vi "Shutdown Frame Grabber.vi"(8 "error in (no error)":errorcluster, 10 "Frame grabber connected?":bool, 11 "Frame Grabber Data in":T1={"Camera Session"="", "Frame"=refnum, "AVI Refnum"=refnum, "Codecs"=[], "Frame number"=0, "Tracking File Refnum"=refnum, "Tick Count"=0, "Probe Object"=refnum, "Playback Probe Data"=[], "Rigid Body"={"Position"={"x (mm)"=0.0, "y (mm)"=0.0, "z (mm)"=0.0}, "Orientation"={"Pitch (rad)"=0.0, "Yaw (rad)"=0.0, "Roll (rad)"=0.0}, "Quaternion"={"qx"=0.0, "qy"=0.0, "qz"=0.0, "qw"=0.0}, "Tracked?"=FALSE}, "Total no frames playback"=0, "Video FPS"=0.0, "Camera connected?"=FALSE, "Scene"=refnum, "Cropped Frame"=refnum, "Tracker FPS"=0.0, "Crop ROI"=[], "Presentation Values"=[], "Elapsed time (ms)"=0, "Camera frames playback"=0, "Refnums"={"Live Refnum"=refnum, "Record Refnum"=refnum, "Recording Settings Refnum"=refnum, "Playback Refnum"=refnum, "Frame Slider Refnum"=refnum, "Pause Refnum"=refnum, "Home Refnum"=refnum, "Crop Refnum"=refnum, "Clear Crop Refnum"=refnum, "stop refnum"=refnum, "Playback Rate Refnum"=refnum, "Operator Settings Refnums"=refnum, "Presentation Refnum"=refnum, "Gestation Refnum"=refnum, "Connection Settings Refnum"=refnum, "Crop Time Frame Slider Refnum"=refnum, "Cancel Save Refnum"=refnum, "Reverse Playback Refnum"=refnum}, "Dimensions"={"Probe Dimensions"={"Probe Width"=0.0, "Probe Depth"=1.0, "Probe Height"=0.0}, "Room Dimensions"={"Room Width"=0.0, "Room Depth"=0.0, "Room Height"=0.0}}, "Playback Data As Strings"=[], "Cropped Tracking File Refnum"=refnum, "Cropped AVI Refnum"=refnum, "Header"=[], "Total euclidian distance"=0.0}) -> (0 "error out":errorcluster, 2 "Disconnect":bool, 3 "Frame Grabber Data out":T1={"Camera Session"="", "Frame"=refnum, "AVI Refnum"=refnum, "Codecs"=[], "Frame number"=0, "Tracking File Refnum"=refnum, "Tick Count"=0, "Probe Object"=refnum, "Playback Probe Data"=[], "Rigid Body"={"Position"={"x (mm)"=0.0, "y (mm)"=0.0, "z (mm)"=0.0}, "Orientation"={"Pitch (rad)"=0.0, "Yaw (rad)"=0.0, "Roll (rad)"=0.0}, "Quaternion"={"qx"=0.0, "qy"=0.0, "qz"=0.0, "qw"=0.0}, "Tracked?"=FALSE}, "Total no frames playback"=0, "Video FPS"=0.0, "Camera connected?"=FALSE, "Scene"=refnum, "Cropped Frame"=refnum, "Tracker FPS"=0.0, "Crop ROI"=[], "Presentation Values"=[], "Elapsed time (ms)"=0, "Camera frames playback"=0, "Refnums"={"Live Refnum"=refnum, "Record Refnum"=refnum, "Recording Settings Refnum"=refnum, "Playback Refnum"=refnum, "Frame Slider Refnum"=refnum, "Pause Refnum"=refnum, "Home Refnum"=refnum, "Crop Refnum"=refnum, "Clear Crop Refnum"=refnum, "stop refnum"=refnum, "Playback Rate Refnum"=refnum, "Operator Settings Refnums"=refnum, "Presentation Refnum"=refnum, "Gestation Refnum"=refnum, "Connection Settings Refnum"=refnum, "Crop Time Frame Slider Refnum"=refnum, "Cancel Save Refnum"=refnum, "Reverse Playback Refnum"=refnum}, "Dimensions"={"Probe Dimensions"={"Probe Width"=0.0, "Probe Depth"=1.0, "Probe Height"=0.0}, "Room Dimensions"={"Room Width"=0.0, "Room Depth"=0.0, "Room Height"=0.0}}, "Playback Data As Strings"=[], "Cropped Tracking File Refnum"=refnum, "Cropped AVI Refnum"=refnum, "Header"=[], "Total euclidian distance"=0.0})   [LabVIEW 2017]
uses:
  Controls/Frame Grabber Data.ctl
  <vilib>/userdefined/High Color/IMAQdx.ctl
  <vilib>/vision/Image Controls.llb/IMAQ Image.ctl
  <vilib>/vision/Avi.llb/IMAQ AVI2 Refnum.ctl
  Controls/Rigid Body Info.ctl
  Controls/Position.ctl
  Controls/Orientation.ctl
  Controls/Refnums.ctl
  Controls/Recording Settings.ctl
  Controls/Operator Settings.ctl
  Controls/Operator.ctl
  Controls/Dimensions.ctl
  Controls/Room Dimensions.ctl
  <vilib>/vision/driver/NI_Vision_Acquisition_Software.lvlib
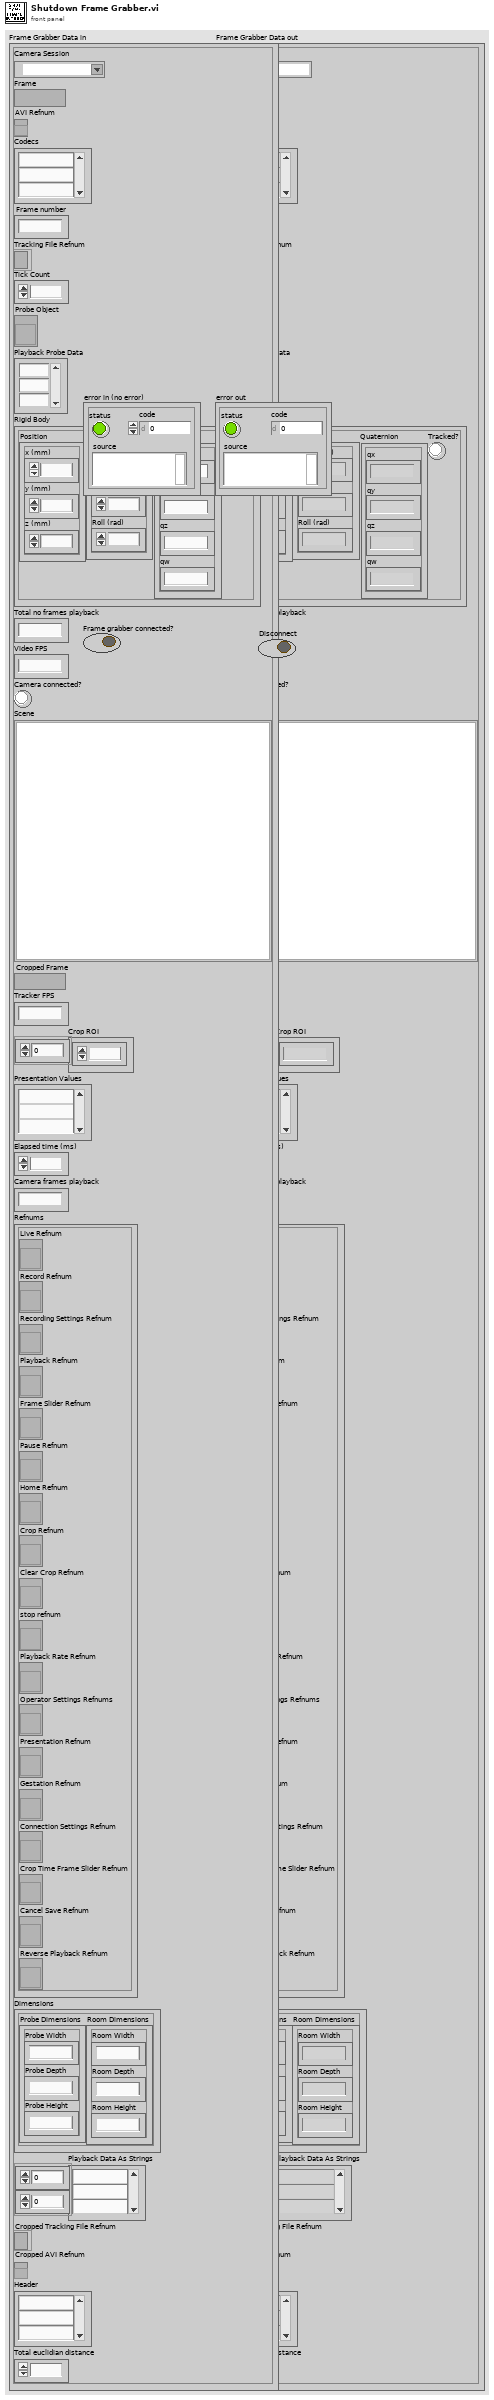
[diagram p1: front panel]
types:
  T1 = typedef "Frame Grabber Data.ctl" = cluster{"Camera Session":T2, "Frame":T3, "AVI Refnum":T4, "Codecs":string[], "Frame number":u32, "Tracking File Refnum":refnum<file>, "Tick Count":u32, "Probe Object":refnum<vi>, "Playback Probe Data":dbl[][], "Rigid Body":T5, "Total no frames playback":i32, "Video FPS":dbl, "Camera connected?":bool, "Scene":refnum<vi>, "Cropped Frame":T3, "Tracker FPS":dbl, "Crop ROI":i32[], "Presentation Values":string[], "Elapsed time (ms)":u32, "Camera frames playback":u32, "Refnums":T8, "Dimensions":T9, "Playback Data As Strings":string[][], "Cropped Tracking File Refnum":refnum<file>, "Cropped AVI Refnum":T4, "Header":string[], "Total euclidian distance":dbl}
  T2 = typedef "IMAQdx.ctl" = refnum<k21>
  T3 = typedef "IMAQ Image.ctl" = refnum<image>
  T4 = typedef "IMAQ AVI2 Refnum.ctl" = refnum<k20>
  T5 = typedef "Rigid Body Info.ctl" = cluster{"Position":T6, "Orientation":T7, "Quaternion":cluster{"qx":sgl, "qy":sgl, "qz":sgl, "qw":sgl}, "Tracked?":bool}
  T6 = typedef "Position.ctl" = cluster{"x (mm)":sgl, "y (mm)":sgl, "z (mm)":sgl}
  T7 = typedef "Orientation.ctl" = cluster{"Pitch (rad)":sgl, "Yaw (rad)":sgl, "Roll (rad)":sgl}
  T8 = typedef "Refnums.ctl" = cluster{"Live Refnum":refnum<vi>, "Record Refnum":refnum<vi>, "Recording Settings Refnum":refnum<vi>, "Playback Refnum":refnum<vi>, "Frame Slider Refnum":refnum<vi>, "Pause Refnum":refnum<vi>, "Home Refnum":refnum<vi>, "Crop Refnum":refnum<vi>, "Clear Crop Refnum":refnum<vi>, "stop refnum":refnum<vi>, "Playback Rate Refnum":refnum<vi>, "Operator Settings Refnums":refnum<vi>, "Presentation Refnum":refnum<vi>, "Gestation Refnum":refnum<vi>, "Connection Settings Refnum":refnum<vi>, "Crop Time Frame Slider Refnum":refnum<vi>, "Cancel Save Refnum":refnum<vi>, "Reverse Playback Refnum":refnum<vi>}
  T9 = typedef "Dimensions.ctl" = cluster{"Probe Dimensions":cluster{"Probe Width":sgl, "Probe Depth":sgl, "Probe Height":sgl}, "Room Dimensions":T10}
  T10 = typedef "Room Dimensions.ctl" = cluster{"Room Width":dbl, "Room Depth":dbl, "Room Height":dbl}
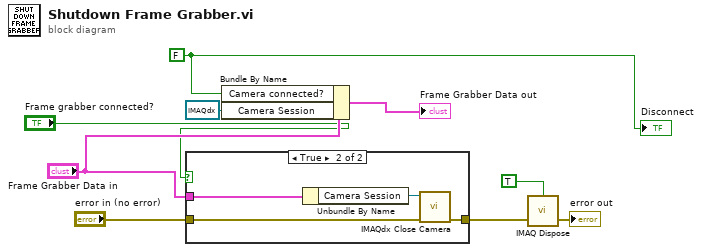
[diagram p0: block diagram]
diagram:
  w1 = FALSE
  n1 = case shown="True" "Frame grabber connected?" {
    tunnel: "Frame Grabber Data in" -> [_ w14]
    tunnel: [w10 w13] -> w5
    tunnel: "error in (no error)" -> [w10 w12]
    frame False {
    }
    frame True {
      n2 = Unbundle By Name(w14) -> ("Camera Session"=w11:T2)
      n3 = call <vilib>:"IMAQdx Close Camera.vi"("error in"=w12, "Session In"=w11) -> ("error out"=w13:errorcluster)  [unwired: 9 in]
    }
  }
  n4 = Bundle By Name(cluster="Frame Grabber Data in", "Camera connected?"=w1, "Camera Session"=T2 refnum) -> (→"Frame Grabber Data out":T1)
  n5 = call "IMAQ Dispose"("All Images? (No)"=TRUE, "error in (no error)"=w5) -> ("error out"=→"error out":errorcluster)  [unwired: 4 in]
  "Disconnect" <- w1
